vi "Idler.vi"(8 "Mission Array In":refnum<class "GenericMission.lvclass">[](array[class]), 9 "BoatLocation":refnum<notifier>, 11 "currently idling?":bool=TRUE) -> (0 "Mission Array out":refnum<class "GenericMission.lvclass">[](array[class]), 3 "still idling?":bool=TRUE)   [LabVIEW 2013]
doc: "Detects when the boat should be in idle mode and implements an idle mission.\n\nKaitlin 4/23"
uses:
  Classes/Missions/GenericMission/GenericMission.lvclass
  Data/TypeDefs/UTM Location.ctl
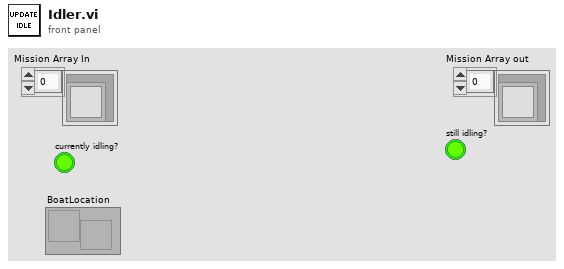
[diagram p1: front panel]
types:
  T1 = typedef "UTM Location.ctl" = cluster{"UTM Zone":dbl, "Hemisphere":enum16{"North", "South"}, "East":dbl, "North":dbl}
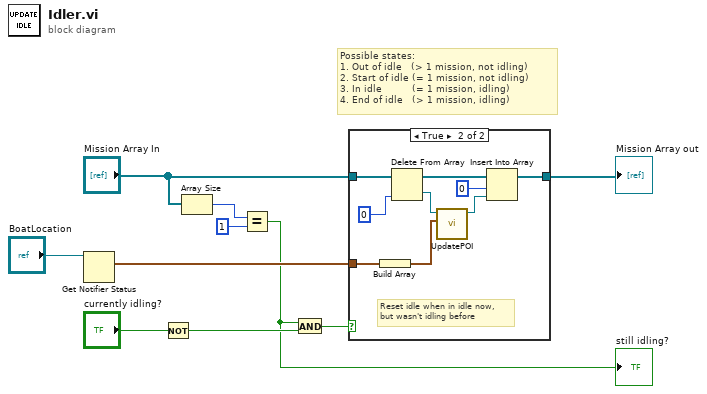
[diagram p0: block diagram]
diagram:
  # "Possible states:\n1. Out of idle   (> 1 mission, not idling)\n2. Start of idle (= 1 mission, not idling)\n3. In idle          (= 1 mission, idling)\n4. End of idle   (> 1 mission, idling)"
  n1 = Get Notifier Status(notifier="BoatLocation") -> (current notification=w5:T1)  [unwired: 1 in, 4 out]
  n2 = Not(x="currently idling?") -> (.not. x?=w2:bool)
  n3 = Array Size(array="Mission Array In") -> (size(s)=w10:i32)
  n4 = Equal?(x=w10, y=1) -> (x = y?=w1:bool)
  "still idling?" <- w1
  n5 = And(x=w1, y=w2) -> (x .and. y?=w3:bool)
  n6 = case shown="True" w3 {
    tunnel: "Mission Array In" -> [w11 w15]
    tunnel: [w11 w20] -> w7
    tunnel: w5 -> [_ w16]
    frame False {
    }
    frame True {
      # "Reset idle when in idle now,\nbut wasn't idling before"
      n7 = Build Array(w16) -> (w17:T1[])
      n8 = Delete From Array(array=w15, index=0) -> (deleted portion=w12:refnum<class "GenericMission.lvclass">, array with subset deleted=w14:refnum<class "GenericMission.lvclass">[])  [unwired: 1 in]
      n9 = call-dynamic "UpdatePOI.vi"("Points of Interest"=w17, "GenericMission in"=w12) -> ("GenericMission out"=w19:refnum<class "GenericMission.lvclass">)  [unwired: 8 in, 1 out]
      n10 = Insert Into Array(array=w14, index=0, new element=w19) -> (w20:refnum<class "GenericMission.lvclass">[])
    }
  }
  "Mission Array out" <- w7
